vi "practice 2.vi"() -> ()   [LabVIEW 2018]
panel:
  out "配列 2":dbl[][](array[numeric])
  out "配列":dbl[](array[numeric])
  out "数値":dbl
  out "ブール":bool
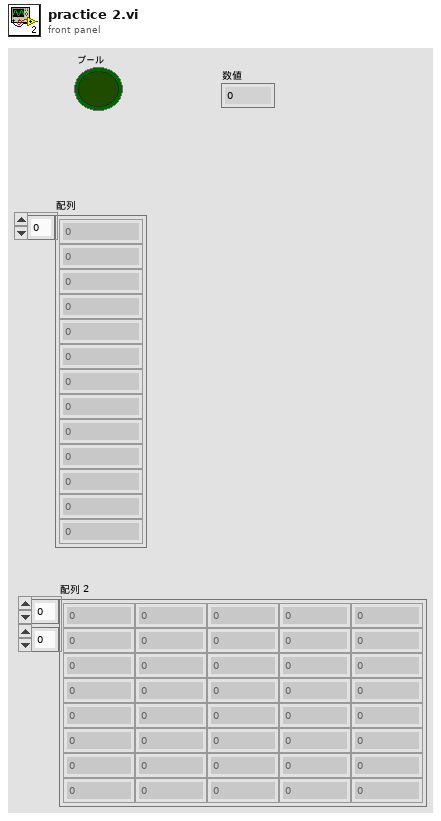
[diagram p1: front panel]
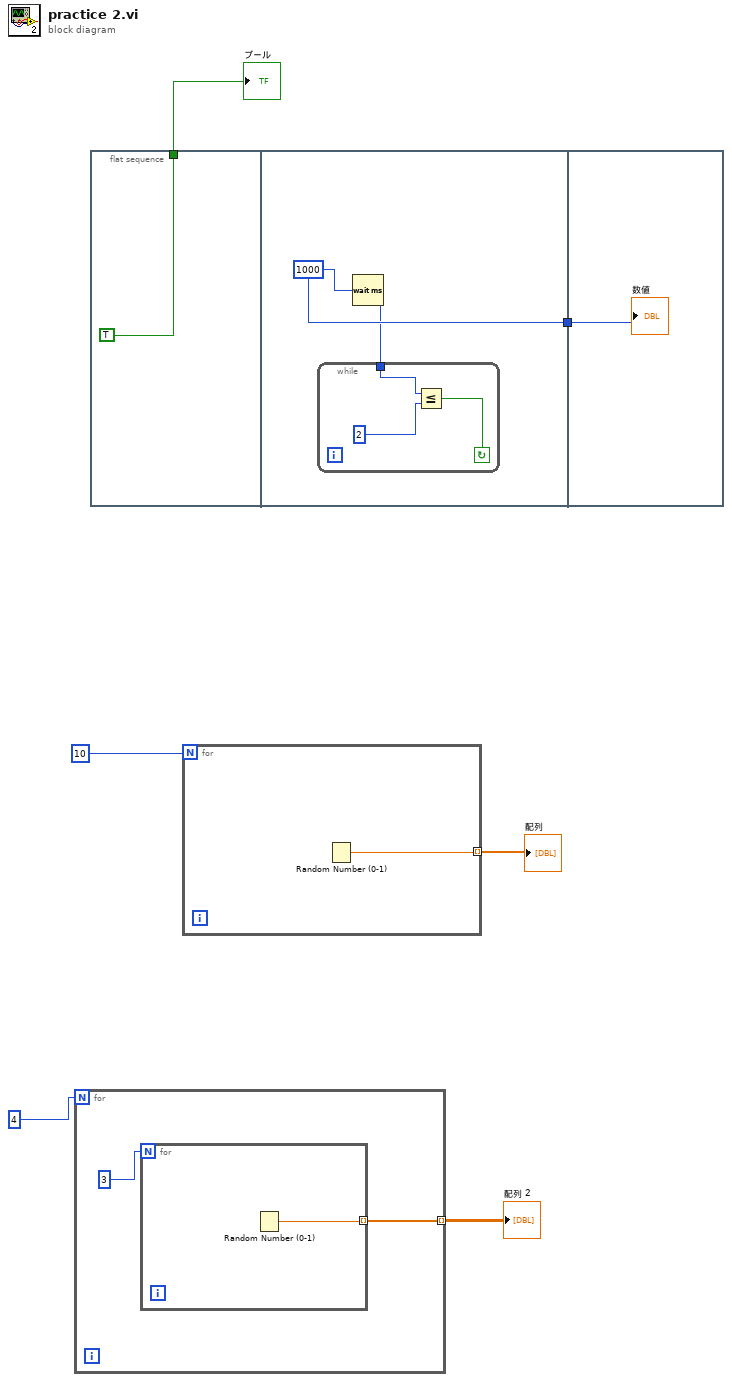
[diagram p0: block diagram]
diagram:
  n1 = for {
    N: 4 -> [_]
    tunnel: [w7] -> w1 mode=indexing
    n2 = for {
      N: 3 -> [_]
      tunnel: [w9] -> w7 mode=indexing
      n3 = Random Number (0-1)() -> (number: 0 to 1=w9:dbl)
    }
  }
  "配列 2" <- w1
  n4 = flat-sequence {
    tunnel: [TRUE] -> w6
    tunnel: [w12] -> w5
    tunnel: w5 -> [w16]
    frame #0 {
    }
    frame #1 {
      w12 = 1000
      n5 = Wait (ms)(milliseconds to wait=w12) -> (millisecond timer value=w11:u32)
      n6 = while {
        tunnel: w11 -> [w14]
        stop <- w15 continue-if-true
        n7 = Less Or Equal?(x=w14, y=2) -> (x <= y?=w15:bool)
      }
    }
    frame #2 {
      "数値" <- w16
    }
  }
  n8 = for {
    N: 10 -> [_]
    tunnel: [w17] -> w3 mode=indexing
    n9 = Random Number (0-1)() -> (number: 0 to 1=w17:dbl)
  }
  "配列" <- w3
  "ブール" <- w6
